vi "VISA Factory.vi"(8 "error in (no error)":errorcluster, 10 "VISA settings":T1) -> (0 "error out":errorcluster, 3 "VISA out":refnum<class "VISA.lvclass">)   [LabVIEW 2018, in "Protocols.lvlib" / "VISA.lvclass"]
doc: "Instantiates a new VISA Protocol object using the provided VISA settings."
uses:
  VISA.lvclass
  VISA Settings.ctl
  VISA.lvclass/VISA.ctl
  Data Access/Write VISA Resource.vi
  Data Access/Write Enable Termination Character.vi
  Data Access/Write Termination Character.vi
  Data Access/Write Timeout.vi
  Data Access/Write Append Write Termination Character.vi
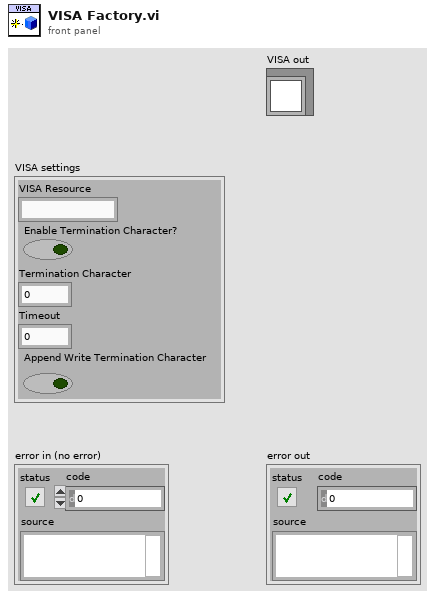
[diagram p1: front panel]
types:
  T1 = typedef "Protocols.lvlib/VISA.lvclass/VISA Settings.ctl" = cluster{"VISA Resource":string, "Enable Termination Character?":bool, "Termination Character":u8, "Timeout":u32, "Append Write Termination Character":bool}
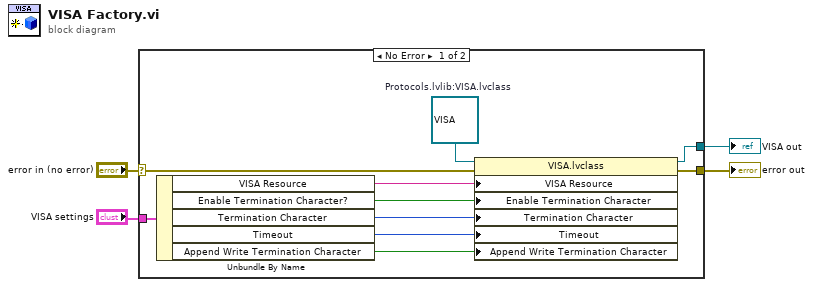
[diagram p0: block diagram]
diagram:
  n1 = case shown="No Error" "error in (no error)" {
    selector: "error in (no error)" -> [w5 w15]
    tunnel: "VISA settings" -> [w14 _]
    tunnel: [w7 _] -> w3
    tunnel: [w6 w15] -> w2
    frame No Error {
      w13 = refnum<class "VISA.lvclass"> refnum  # Protocols.lvlib:VISA.lvclass
      n2 = Unbundle By Name(w14) -> ("VISA Resource"=w12:string, "Enable Termination Character?"=w11:bool, "Termination Character"=w10:u8, "Timeout"=w9:u32, "Append Write Termination Character"=w8:bool)
      n3 = property class="VISA.lvclass"(reference=w13, error in=w5, "VISA Resource"=w12, "Enable Termination Character"=w11, "Termination Character"=w10, "Timeout"=w9, "Append Write Termination Character"=w8) -> (reference out=w7:refnum<class "VISA.lvclass">, error out=w6:errorcluster)
    }
    frame Error {
    }
  }
  "VISA out" <- w3
  "error out" <- w2
